vi "punto_2.vi"() -> ()   [LabVIEW 2018]
panel:
  in  "stop":bool
  in  "Acción":bool
  in  "Llenado/Vaciado":bool
  in  "Velocidad":bool
  out "Tanque Vacio":bool
  out "Tanque Lleno":bool
  out "Paro":bool
  out "Llenando":bool
  out "Vaciando":bool
  out "Tanque":dbl(slide) scale=0.0..1000.0
  # "Alta"
  # "Baja"
  # "continuar"
  # "Parar"
  # "Llenar"
  # "Vaciar"
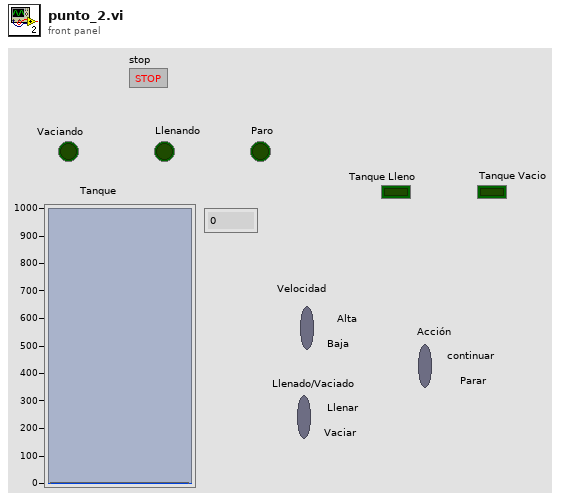
[diagram p1: front panel]
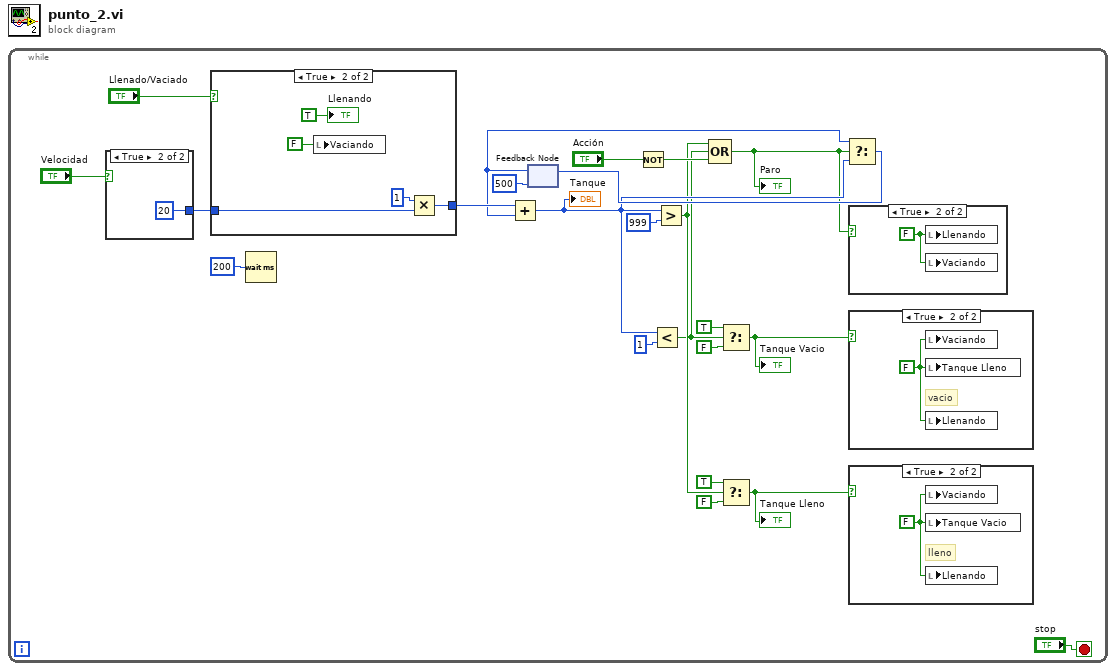
[diagram p0: block diagram]
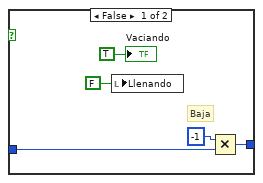
[diagram p5: hidden frame]
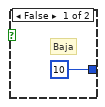
[diagram p6: hidden frame]
diagram:
  n1 = while {
    stop <- "stop" stop-if-true
    n2 = case shown="True" "Velocidad" {
      tunnel: [10 20] -> w19
      frame False {
        # "Baja"
      }
      frame True {
      }
    }
    n3 = case shown="True" "Llenado/Vaciado" {
      tunnel: w19 -> [w30 w36]
      tunnel: [w29 w34] -> w17
      frame False {
        # "Baja"
        n4 = local write "Llenando"(FALSE ("Llenando")) -> ()
        n5 = Multiply(x=-1, y=w30) -> (x*y=w29:i32)
        "Vaciando" <- TRUE ("Vaciando")
      }
      frame True {
        n6 = local write "Vaciando"(FALSE ("Vaciando")) -> ()
        n7 = Multiply(x=1 ("y"), y=w36) -> (x*y=w34:i32)
        "Llenando" <- TRUE ("Llenando")
      }
    }
    n8 = Wait (ms)(milliseconds to wait=u32 200) -> ()  [unwired: 1 out]
    n9 = feedback #1(500) -> (w13:i32)
    n10 = Add(x=w17, y=w13) -> (x+y=w12:i32)
    "Tanque" <- w12
    n11 = Not(x="Acción") -> (.not. x?=w11:bool)
    n12 = Less?(x=w12, y=1) -> (x < y?=w3:bool)
    n13 = Greater?(x=w12, y=999) -> (0:w9:bool)
    n14 = Compound Arithmetic op=OR(w9, w3, w11) -> (w1:bool)
    "Paro" <- w1
    n15 = Select(t=TRUE ("Tanque Vacio"), s=w3, f=FALSE ("Tanque Vacio")) -> (s? t:f=w2:bool)
    "Tanque Vacio" <- w2
    n16 = Select(t=TRUE ("Tanque Vacio"), s=w9, f=FALSE ("Tanque Vacio")) -> (s? t:f=w6:bool)
    "Tanque Lleno" <- w6
    n17 = Select(t=w13, s=w1, f=w12) -> (s? t:f=w14:i32)
    n18 = feedback-in #1(w14) -> ()
    n19 = case shown="True" w1 {
      frame False {
      }
      frame True {
        w24 = FALSE ("Llenando")
        n20 = local write "Llenando"(w24) -> ()
        n21 = local write "Vaciando"(w24) -> ()
      }
    }
    n22 = case shown="True" w2 {
      frame False {
      }
      frame True {
        w26 = FALSE ("Llenando")
        # "vacio"
        n23 = local write "Vaciando"(w26) -> ()
        n24 = local write "Tanque Lleno"(w26) -> ()
        n25 = local write "Llenando"(w26) -> ()
      }
    }
    n26 = case shown="True" w6 {
      frame False {
      }
      frame True {
        w25 = FALSE ("Llenando")
        # "lleno"
        n27 = local write "Vaciando"(w25) -> ()
        n28 = local write "Tanque Vacio"(w25) -> ()
        n29 = local write "Llenando"(w25) -> ()
      }
    }
  }
